vi "Capture_Save_Initialize.vi"(11 "input cluster":T1={"Pinch-valve"="Test Sample", "XLP 6000 Pump"="MRJ", "Camera1"="", "Camera2"="", "Img_Capt"=FALSE, "Actuator"=FALSE, "Pump"=FALSE, "Cam 1"=FALSE, "Cam 2"=FALSE, "Empty_Refill"=FALSE, "Crop"=FALSE, "Light intensity"=0, "Exposure Time"=0.0, "Sample Name"="", "Operator"="", "Calibration 1"=path "C:/Users/au540322/Desktop/IHS_Project/images/Debris/Debris_0/Debris_0_2019_06_01-23-32-49-686.PNG", "Calibration 2"=path "C:/Users/au540322/Desktop/IHS_Project/images/Debris/Debris_0/Debris_0_2019_06_01-23-32-49-686.PNG", "Framerate"=1, "Timeout Sample"=1, "Collection date"="", "Sample size threshold"=500, "Empty start"=500, "Command"="", "Station"="", "Species Name"="", "Other Notes"="", "Aperture"=enum."Item 3", "Image Process Queue Size"=100, "Image Save Queue Size"=0, "Overload threshold"=0, "Max Framerate"=0, "Rectangle 1"={"Left"=0, "Top"=0, "Right"=0, "Bottom"=0, "Rotation"=0.0}, "Rectangle 2"={"Left"=0, "Top"=100, "Right"=100, "Bottom"=0, "Rotation"=0.0}, "Detection Region %"=200.0, "Detect 1"=path "C:/Users/au540322/Desktop/IHS_Project/images/Debris/Debris_0/Debris_0_2019_06_01-23-32-49-686.PNG", "Detect 2"=path "C:/Users/au540322/Desktop/IHS_Project/images/Debris/Debris_0/Debris_0_2019_06_01-23-32-49-686.PNG", "Max large object threshold"=500, "Open(T)/Close(F)"=FALSE, "Img_Capt Begin"=FALSE, "Dispense Speed"=0, "Flush Size"=0, "Location"="", "Latitude"="", "Longitude"="", "Determiner"="", "Sex"="", "Camera1_Img"=refnum, "Camera2_Img"=refnum, "Img1_Orig_Disp"=refnum, "Img2_Orig_Disp"=refnum, "Img1_Orig_RGB"=refnum, "Img2_Orig_RGB"=refnum, "Blue_Plane_Extract"=refnum, "Subtracted_Plane"=refnum, "Img1_Binary"=refnum, "Img2_Binary"=refnum, "Crop_Mask"=refnum, "Img1_Save"=refnum, "Img2_Save"=refnum, "Img1_Cali_Full"=refnum, "Img2_Cali_Full"=refnum, "Img1_Cali_Detect"=refnum, "Img2_Cali_Detect"=refnum, "Cam 1 queue"=refnum, "Cam 2 queue"=refnum, "Cam 1 - save queue"=refnum, "Cam 2 - save queue"=refnum, "Overlay_Ring"=0, "SystemVersion"=0, "System Serial"="", "Legacy Cam Attributes"=FALSE, "Camera Orientation 1"="", "Camera Orientation 2"="", "Pixel to mm 1"=0.0, "Pixel to mm 2"=0.0, "CAM1 Model"=enum."a2A5328-15ucBAS", "CAM2 Model"=enum."a2A5328-15ucBAS", "Flush Insect"=FALSE, "Pump Size"=FALSE, "Barcode"="", "Phase3"=FALSE, "Mega F3"="", "Container nr."=0.0, "Flush Error"=TRUE, "Start System"=FALSE, "Size Interval"=0.0, "Mun. of containers"=0.0, "Sorting sys."=FALSE, "Initial size"=0.0} {"SystemVersion" items=["Standard", "XL"]; "Overlay_Ring" items=["Session Data", "Extended Setup", "Buffer", "Camera", "Dispenser", "Stats", "Connections"]; "Flush Size" min=1; "Dispense Speed" min=1; "Rectangle 2"."Rotation" format="%.2f"; "Rectangle 2"."Left" scale=0.0..1024.0; "Rectangle 2"."Right" scale=0.0..1024.0; "Rectangle 1"."Rotation" format="%.2f"; "Rectangle 1"."Left" scale=0.0..1024.0; "Rectangle 1"."Right" scale=0.0..1024.0; "Max Framerate" min=1; "Overload threshold" min=1; "Image Save Queue Size" min=1; "Image Process Queue Size" min=1; "Empty start" min=1; "Sample size threshold" min=1; "Framerate" min=1; "Light intensity" scale=0.0..100.0}) -> (3 "output cluster":T1={"Pinch-valve"="Test Sample", "XLP 6000 Pump"="MRJ", "Camera1"="", "Camera2"="", "Img_Capt"=FALSE, "Actuator"=FALSE, "Pump"=FALSE, "Cam 1"=FALSE, "Cam 2"=FALSE, "Empty_Refill"=FALSE, "Crop"=FALSE, "Light intensity"=0, "Exposure Time"=0.0, "Sample Name"="", "Operator"="", "Calibration 1"=path "C:/Users/au540322/Desktop/IHS_Project/images/Debris/Debris_0/Debris_0_2019_06_01-23-32-49-686.PNG", "Calibration 2"=path "C:/Users/au540322/Desktop/IHS_Project/images/Debris/Debris_0/Debris_0_2019_06_01-23-32-49-686.PNG", "Framerate"=100, "Timeout Sample"=500, "Collection date"="", "Sample size threshold"=500, "Empty start"=500, "Command"="", "Station"="", "Species Name"="", "Other Notes"="", "Aperture"=enum."Item 3", "Image Process Queue Size"=100, "Image Save Queue Size"=0, "Overload threshold"=0, "Max Framerate"=0, "Rectangle 1"={"Left"=0, "Top"=0, "Right"=0, "Bottom"=0, "Rotation"=0.0}, "Rectangle 2"={"Left"=0, "Top"=100, "Right"=100, "Bottom"=0, "Rotation"=0.0}, "Detection Region %"=200.0, "Detect 1"=path "C:/Users/au540322/Desktop/IHS_Project/images/Debris/Debris_0/Debris_0_2019_06_01-23-32-49-686.PNG", "Detect 2"=path "C:/Users/au540322/Desktop/IHS_Project/images/Debris/Debris_0/Debris_0_2019_06_01-23-32-49-686.PNG", "Max large object threshold"=500, "Open(T)/Close(F)"=FALSE, "Img_Capt Begin"=FALSE, "Dispense Speed"=0, "Flush Size"=0, "Location"="", "Latitude"="", "Longitude"="", "Determiner"="", "Sex"="", "Camera1_Img"=refnum, "Camera2_Img"=refnum, "Img1_Orig_Disp"=refnum, "Img2_Orig_Disp"=refnum, "Img1_Orig_RGB"=refnum, "Img2_Orig_RGB"=refnum, "Blue_Plane_Extract"=refnum, "Subtracted_Plane"=refnum, "Img1_Binary"=refnum, "Img2_Binary"=refnum, "Crop_Mask"=refnum, "Img1_Save"=refnum, "Img2_Save"=refnum, "Img1_Cali_Full"=refnum, "Img2_Cali_Full"=refnum, "Img1_Cali_Detect"=refnum, "Img2_Cali_Detect"=refnum, "Cam 1 queue"=refnum, "Cam 2 queue"=refnum, "Cam 1 - save queue"=refnum, "Cam 2 - save queue"=refnum, "Overlay_Ring"=0, "SystemVersion"=0, "System Serial"="", "Legacy Cam Attributes"=FALSE, "Camera Orientation 1"="", "Camera Orientation 2"="", "Pixel to mm 1"=0.0, "Pixel to mm 2"=0.0, "CAM1 Model"=enum."a2A5328-15ucBAS", "CAM2 Model"=enum."a2A5328-15ucBAS", "Flush Insect"=FALSE, "Pump Size"=FALSE, "Barcode"="", "Phase3"=FALSE, "Mega F3"="", "Container nr."=0.0, "Flush Error"=TRUE, "Start System"=FALSE, "Size Interval"=0.0, "Mun. of containers"=0.0, "Sorting sys."=FALSE, "Initial size"=0.0} {"SystemVersion" items=["Standard", "XL"]; "Overlay_Ring" items=["Session Data", "Extended Setup", "Buffer", "Camera", "Dispenser", "Stats", "Connections"]; "Flush Size" min=1; "Dispense Speed" min=1; "Rectangle 2"."Rotation" format="%.2f"; "Rectangle 2"."Left" scale=0.0..1024.0; "Rectangle 2"."Right" scale=0.0..1024.0; "Rectangle 1"."Rotation" format="%.2f"; "Rectangle 1"."Left" scale=0.0..1024.0; "Rectangle 1"."Right" scale=0.0..1024.0; "Max Framerate" min=1; "Overload threshold" min=1; "Image Save Queue Size" min=1; "Image Process Queue Size" min=1; "Empty start" min=1; "Sample size threshold" min=1; "Framerate" min=1; "Light intensity" scale=0.0..100.0})   [LabVIEW 2024]
uses:
  controls/Data.ctl
  <vilib>/userDefined/High Color/IMAQdx.ctl
  <vilib>/vision/Image Controls.llb/IMAQ Image.ctl
  <vilib>/vision/driver/IMAQdx.llb/IMAQdx Acquisition Mode.ctl
  <vilib>/vision/driver/NI_Vision_Acquisition_Software.lvlib
types:
  T1 = typedef "Data.ctl" = cluster{"Pinch-valve":refnum<visa-resource-name>, "XLP 6000 Pump":refnum<visa-resource-name>, "Camera1":T2, "Camera2":T2, "Img_Capt":bool, "Actuator":bool, "Pump":bool, "Cam 1":bool, "Cam 2":bool, "Empty_Refill":bool, "Crop":bool, "Light intensity":i32, "Exposure Time":dbl, "Sample Name":string, "Operator":string, "Calibration 1":path, "Calibration 2":path, "Framerate":i32, "Timeout Sample":i32, "Collection date":string, "Sample size threshold":i32, "Empty start":u32, "Command":string, "Station":string, "Species Name":string, "Other Notes":string, "Aperture":enum32{"Item 0", "Item 1", "Item 2", "Item 3"}, "Image Process Queue Size":i32, "Image Save Queue Size":i32, "Overload threshold":i32, "Max Framerate":i32, "Rectangle 1":T3, "Rectangle 2":T3, "Detection Region %":dbl, "Detect 1":path, "Detect 2":path, "Max large object threshold":i32, "Open(T)/Close(F)":bool, "Img_Capt Begin":bool, "Dispense Speed":i32, "Flush Size":i32, "Location":string, "Latitude":string, "Longitude":string, "Determiner":string, "Sex":string, "Camera1_Img":T4, "Camera2_Img":T4, "Img1_Orig_Disp":T4, "Img2_Orig_Disp":T4, "Img1_Orig_RGB":T4, "Img2_Orig_RGB":T4, "Blue_Plane_Extract":T4, "Subtracted_Plane":T4, "Img1_Binary":T4, "Img2_Binary":T4, "Crop_Mask":T4, "Img1_Save":T4, "Img2_Save":T4, "Img1_Cali_Full":T4, "Img2_Cali_Full":T4, "Img1_Cali_Detect":T4, "Img2_Cali_Detect":T4, "Cam 1 queue":refnum<queue>, "Cam 2 queue":refnum<queue>, "Cam 1 - save queue":refnum<queue>, "Cam 2 - save queue":refnum<queue>, "Overlay_Ring":u16, "SystemVersion":u16, "System Serial":string, "Legacy Cam Attributes":bool, "Camera Orientation 1":string, "Camera Orientation 2":string, "Pixel to mm 1":dbl, "Pixel to mm 2":dbl, "CAM1 Model":enum16{"a2A5328-15ucBAS", "acA1920-155uc"}, "CAM2 Model":enum16{"a2A5328-15ucBAS", "acA1920-155uc"}, "Flush Insect":bool, "Pump Size":bool, "Barcode":string, "Phase3":bool, "Mega F3":refnum<visa-resource-name>, "Container nr.":dbl, "Flush Error":bool, "Start System":bool, "Size Interval":dbl, "Mun. of containers":dbl, "Sorting sys.":bool, "Initial size":dbl}
  T2 = typedef "IMAQdx.ctl" = refnum<k21>
  T3 = typedef "IMAQ Rectangle" = cluster{"Left":i32, "Top":i32, "Right":i32, "Bottom":i32, "Rotation":dbl}
  T4 = typedef "IMAQ Image.ctl" = refnum<image>
  T5 = typedef "Image Type" = u32
  T6 = cluster{"Timestamp":string, "Image Pixels (U32)":u32[][], "Prev. sample":i32, "Sample Data":dbl[], "output cluster":cluster{"Global Rectangle":i32[], "Contours":cluster{"ID":enum32{"External", "Internal"}, "Type":u32, "Coordinates":i32[]}[]}}
  T7 = cluster{"Image Pixels (U32)":u32[][], "Detect Movement":bool, string}
  T8 = typedef "NI_Vision_Acquisition_Software.lvlib/IMAQdx Acquisition Mode.ctl" = enum32{"One Shot", "Continuous"}
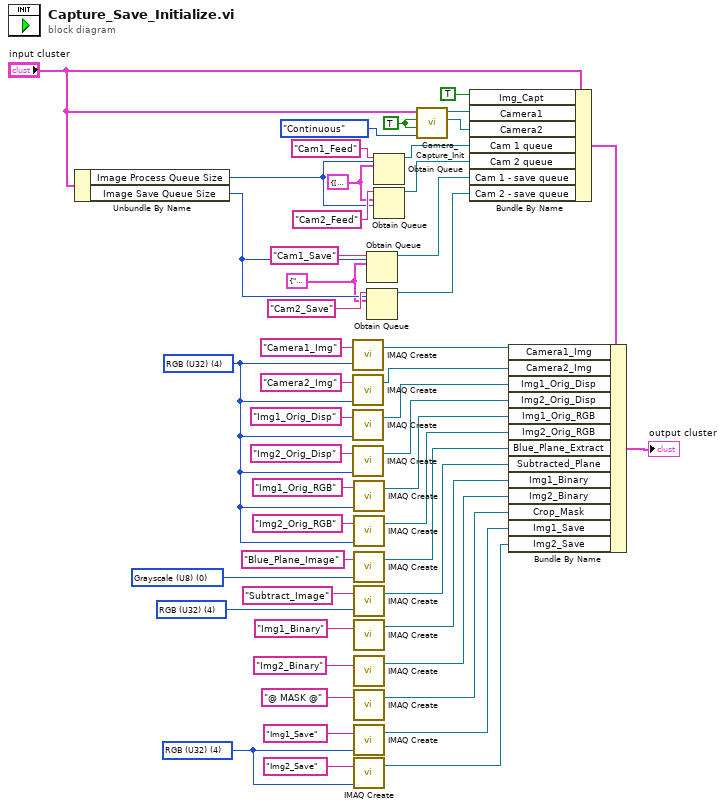
[diagram p0: block diagram]
diagram:
  w1 = T5 0 items=["Grayscale (U8)", "Grayscale (I16)", "Grayscale (SGL)", "Complex (CSG)", "RGB (U32)", "HSL (U32)", "RGB (U64)", "Grayscale (U16)"] ("Image Type")
  w2 = T5 4 items=["Grayscale (U8)", "Grayscale (I16)", "Grayscale (SGL)", "Complex (CSG)", "RGB (U32)", "HSL (U32)", "RGB (U64)", "Grayscale (U16)"] ("Image Type")
  w3 = T6 {"Timestamp"="", "Image Pixels (U32)"=[], "Prev. sample"=0, "Sample Data"=[], "output cluster"={"Global Rectangle"=[], "Contours"=[]}} ("output cluster")
  w4 = T7 {"Image Pixels (U32)"=[], "Detect Movement"=FALSE, ""} ("output cluster")
  w20 = T5 4 items=["Grayscale (U8)", "Grayscale (I16)", "Grayscale (SGL)", "Complex (CSG)", "RGB (U32)", "HSL (U32)", "RGB (U64)", "Grayscale (U16)"] ("Image Type")
  w5 = T5 4 items=["Grayscale (U8)", "Grayscale (I16)", "Grayscale (SGL)", "Complex (CSG)", "RGB (U32)", "HSL (U32)", "RGB (U64)", "Grayscale (U16)"] ("Image Type")
  w25 = TRUE ("Crop?")
  n1 = Unbundle By Name("input cluster") -> ("Image Process Queue Size"=w36:i32, "Image Save Queue Size"=w24:i32)
  n2 = call "IMAQ Create"("Image Name"="Camera1_Img", "Image Type"=w5) -> ("New Image"=w19:T4)  [unwired: 3 in, 1 out]
  n3 = call "IMAQ Create"("Image Name"="Camera2_Img", "Image Type"=w5) -> ("New Image"=w18:T4)  [unwired: 3 in, 1 out]
  n4 = call "IMAQ Create"("Image Name"="Img1_Orig_Disp", "Image Type"=w5) -> ("New Image"=w17:T4)  [unwired: 2 in, 2 out]
  n5 = call "IMAQ Create"("Image Name"="Img2_Orig_Disp", "Image Type"=w5) -> ("New Image"=w16:T4)  [unwired: 2 in, 2 out]
  n6 = call "IMAQ Create"("Image Name"="Img1_Orig_RGB", "Image Type"=w5) -> ("New Image"=w15:T4)  [unwired: 2 in, 2 out]
  n7 = call "IMAQ Create"("Image Name"="Img2_Orig_RGB", "Image Type"=w5) -> ("New Image"=w14:T4)  [unwired: 2 in, 2 out]
  n8 = call "IMAQ Create"("Image Name"="Blue_Plane_Image", "Image Type"=w1) -> ("New Image"=w13:T4)  [unwired: 2 in, 2 out]
  n9 = call "IMAQ Create"("Image Name"="Subtract_Image", "Image Type"=w2) -> ("New Image"=w12:T4)  [unwired: 2 in, 2 out]
  n10 = call "IMAQ Create"("Image Name"="Img1_Binary") -> ("New Image"=w11:T4)  [unwired: 3 in, 2 out]
  n11 = call "IMAQ Create"("Image Name"="Img2_Binary") -> ("New Image"=w10:T4)  [unwired: 3 in, 2 out]
  n12 = call "IMAQ Create"("Image Name"="@ MASK @") -> ("New Image"=w9:T4)  [unwired: 3 in, 2 out]
  n13 = call "IMAQ Create"("Image Name"="Img1_Save", "Image Type"=w20) -> ("New Image"=w8:T4)  [unwired: 2 in, 2 out]
  n14 = call "IMAQ Create"("Image Name"="Img2_Save", "Image Type"=w20) -> ("New Image"=w7:T4)  [unwired: 2 in, 2 out]
  n15 = Obtain Queue(max queue size (-1, unlimited)=w24, name (unnamed)="Cam1_Save", element data type=w3) -> (queue out=w29:refnum<queue>)  [unwired: 2 in, 2 out]
  n16 = Obtain Queue(max queue size (-1, unlimited)=w24, name (unnamed)="Cam2_Save", element data type=w3) -> (queue out=w28:refnum<queue>)  [unwired: 2 in, 2 out]
  n17 = Obtain Queue(max queue size (-1, unlimited)=w36, name (unnamed)="Cam1_Feed", element data type=w4) -> (queue out=w42:refnum<queue>)  [unwired: 2 in, 2 out]
  n18 = Obtain Queue(max queue size (-1, unlimited)=w36, name (unnamed)="Cam2_Feed", element data type=w4) -> (queue out=w41:refnum<queue>)  [unwired: 2 in, 2 out]
  n19 = call "Camera_Capture_Init.vi"("Continuous?"=IMAQdx_Acquisition_Mode."Continuous", "Detect Movement"=w25, "Crop?"=w25, "input cluster"="input cluster") -> ("Camera2"=w46:T2, "Camera1"=w47:T2)  [unwired: 6 in]
  n20 = Bundle By Name(cluster="input cluster", "Img_Capt"=TRUE ("Image_Capture"), "Camera1"=w47, "Camera2"=w46, "Cam 1 queue"=w42, "Cam 2 queue"=w41, "Cam 1 - save queue"=w29, "Cam 2 - save queue"=w28) -> (w23:T1)
  n21 = Bundle By Name(cluster=w23, "Camera1_Img"=w19, "Camera2_Img"=w18, "Img1_Orig_Disp"=w17, "Img2_Orig_Disp"=w16, "Img1_Orig_RGB"=w15, "Img2_Orig_RGB"=w14, "Blue_Plane_Extract"=w13, "Subtracted_Plane"=w12, "Img1_Binary"=w11, "Img2_Binary"=w10, "Crop_Mask"=w9, "Img1_Save"=w8, "Img2_Save"=w7) -> (→"output cluster":T1)
